vi "SelectMonitor.vi"(8 "Error In":errorcluster, 9 "Center?":bool, 10 "Monitor (0=primary)":u16, 11 "VI Ref In":refnum<vi>) -> (0 "Error out":errorcluster, 3 "VI Ref Out":refnum<vi>)   [LabVIEW 2013, in "LV-Utilities.lvlib"]
uses:
  LV-Utilities.lvlib
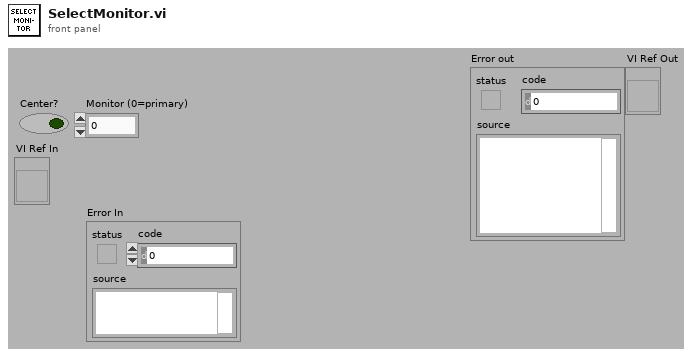
[diagram p1: front panel]
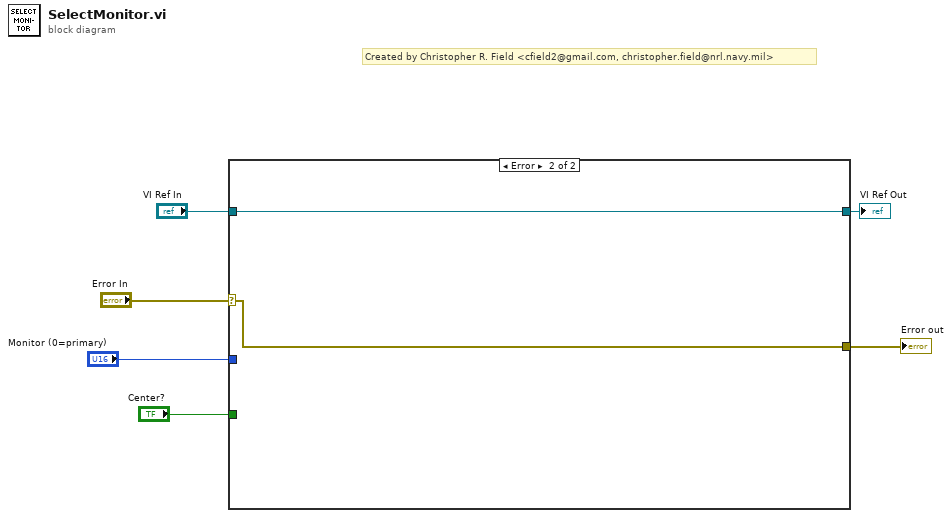
[diagram p0: block diagram]
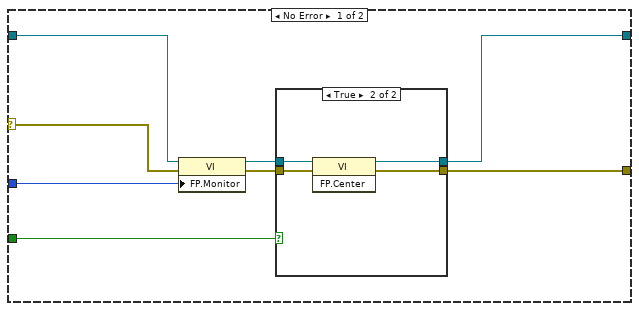
[diagram p2: hidden frame]
diagram:
  # "Created by Christopher R. Field <cfield2@gmail.com, christopher.field@nrl.navy.mil>"
  n1 = case shown="Error" "Error In" {
    selector: "Error In" -> [w9 w22]
    tunnel: [w8 w22] -> w6
    tunnel: "Center?" -> [w12 _]
    tunnel: "Monitor (0=primary)" -> [w11 _]
    tunnel: "VI Ref In" -> [w10 w21]
    tunnel: [w7 w21] -> w1
    frame No Error {
      n2 = property class="VI"(reference=w10, error in=w9, "FP.Monitor"=w11) -> (reference out=w14:refnum<vi>, error out=w13:errorcluster)
      n3 = case shown="True" w12 {
        tunnel: w14 -> [w16 w20]
        tunnel: w13 -> [w15 w19]
        tunnel: [w15 w18] -> w8
        tunnel: [w16 w17] -> w7
        frame False {
        }
        frame True {
          n4 = invoke class="VI" method="FP.Center"(reference=w20, error in=w19) -> (reference out=w17:refnum<vi>, error out=w18:errorcluster)  [unwired: 1 in, 1 out]
        }
      }
    }
    frame Error {
    }
  }
  "Error out" <- w6
  "VI Ref Out" <- w1
